vi "Write 7z bat.vi"(8 "error in (no error)":errorcluster, 9 "Product Name":string, 10 "Package Version":string, 11 "source path":path) -> (0 "error out":errorcluster)   [LabVIEW 2016]
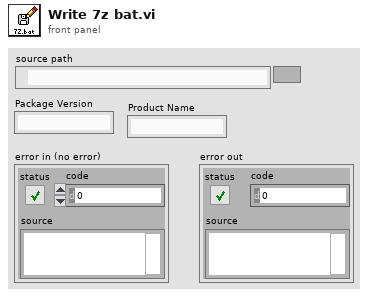
[diagram p1: front panel]
types:
  T1 = enum16{"open", "replace", "create", "open or create", "replace or create", "replace or create with confirmation"}
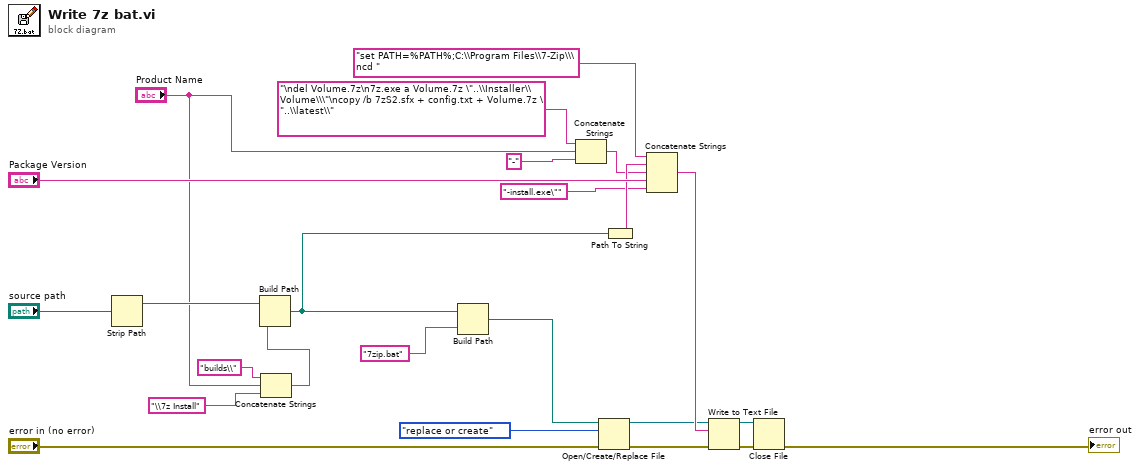
[diagram p0: block diagram]
diagram:
  n1 = Strip Path(path="source path") -> (stripped path=w20:path)  [unwired: 1 out]
  n2 = Concatenate Strings("builds\\" ("name or relative path"), "Product Name", "\\7z Install" ("name or relative path")) -> (w7:string)
  n3 = Build Path(base path=w20, name or relative path=w7) -> (appended path=w10:path)
  n4 = Build Path(base path=w10, name or relative path="7zip.bat") -> (appended path=w17:path)
  n5 = Concatenate Strings("\ndel Volume.7z\n7z.exe a Volume.7z \"..\\Installer\\Volume\\\"\ncopy /b 7zS2.sfx + config.txt + Volume.7z \"..\\latest\\" ("Name of target (My Computer)"), "Product Name", "-" ("Name of target (My Computer)")) -> (w2:string)
  n6 = Open/Create/Replace File(file path (use dialog)=w17, error in="error in (no error)", operation (0:open)=T1."replace or create") -> (refnum out=w18:refnum<file>, error out=w15:errorcluster)  [unwired: 3 in, 1 out]
  n7 = Path To String(path=w10) -> (string=w9:string)
  n8 = Concatenate Strings("set PATH=%PATH%;C:\\Program Files\\7-Zip\\\ncd " ("Name of target (My Computer)"), w9, w2, "Package Version", "-install.exe\"" ("Name of target (My Computer)")) -> (w24:string)
  n9 = Write to Text File(file (use dialog)=w18, text=w24, error in=w15) -> (refnum out=w12:refnum<file>, error out=w13:errorcluster)  [unwired: 1 in, 1 out]
  n10 = Close File(refnum=w12, error in=w13) -> (error out=→"error out":errorcluster)  [unwired: 1 out]
